vi "SaveLEDSettingsToFile.vi"(5 "Prefix":string="LEDSetting", 9 "Save?":bool, 10 "LED Color Ref":refnum<vi>, 11 "name or relative path":string) -> (3 "Saved Settings Path":path)   [LabVIEW 2015]
uses:
  <vilib>/Utility/sysdir.llb/System Directory Type.ctl
  <vilib>/Utility/file.llb/Write Delimited Spreadsheet (string).vi
panel:
  in  "LED Color":T1={"Hue"={110.52399131877658, 148.6727294921875}, "Sat"={34.78571428571429, 255.0}, "Val"={91.07142857142858, 255.0}} {"Hue" scale=0.0..255.0 scale format="%#_3g"}
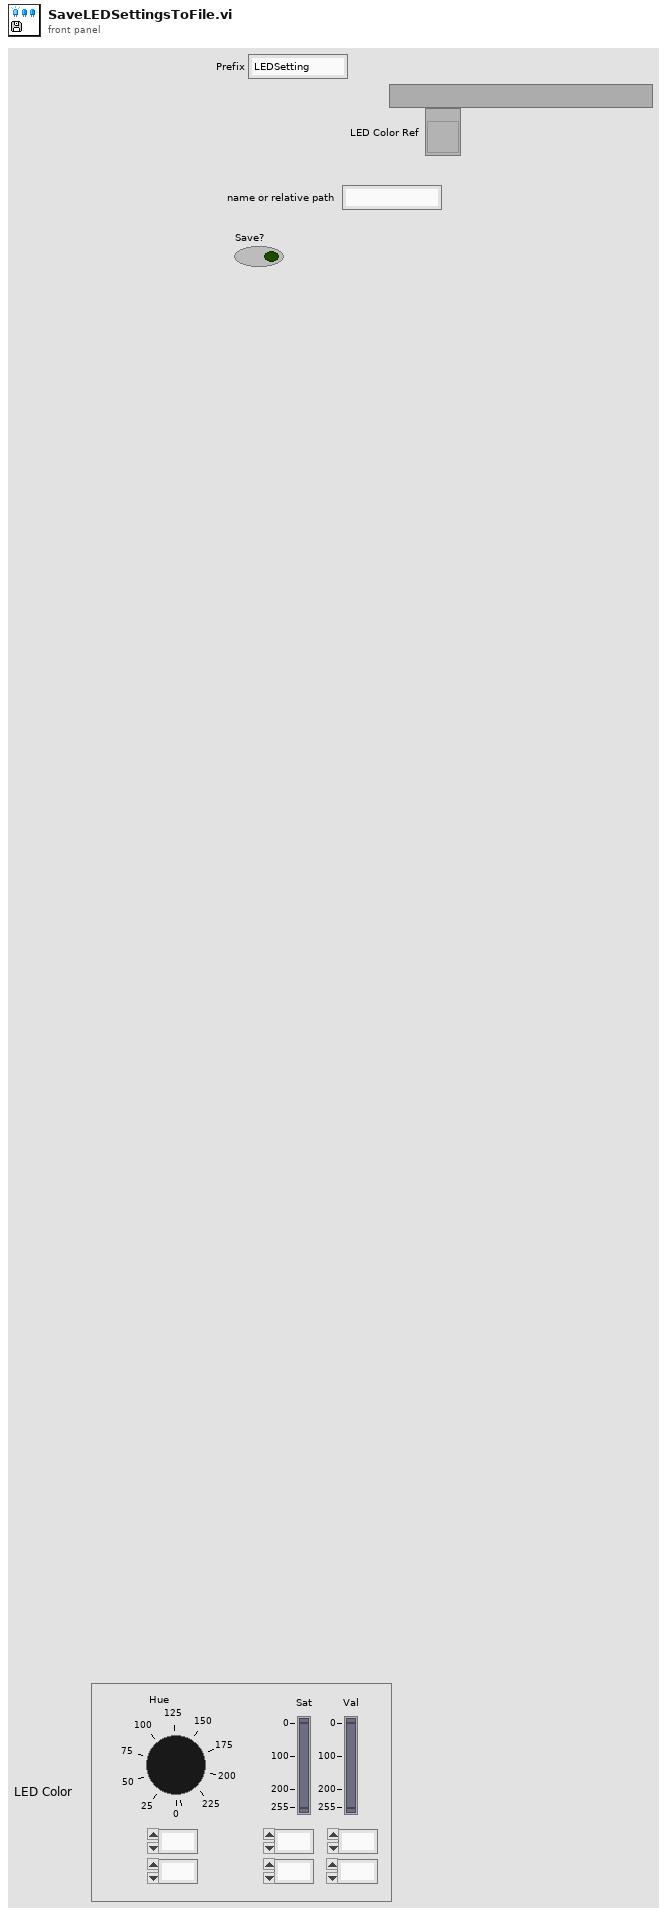
[diagram p1: front panel]
types:
  T1 = cluster{"Hue":cluster{dbl, dbl}, "Sat":cluster{dbl, dbl}, "Val":cluster{dbl, dbl}}
  T2 = typedef "System Directory Type.ctl" = i32
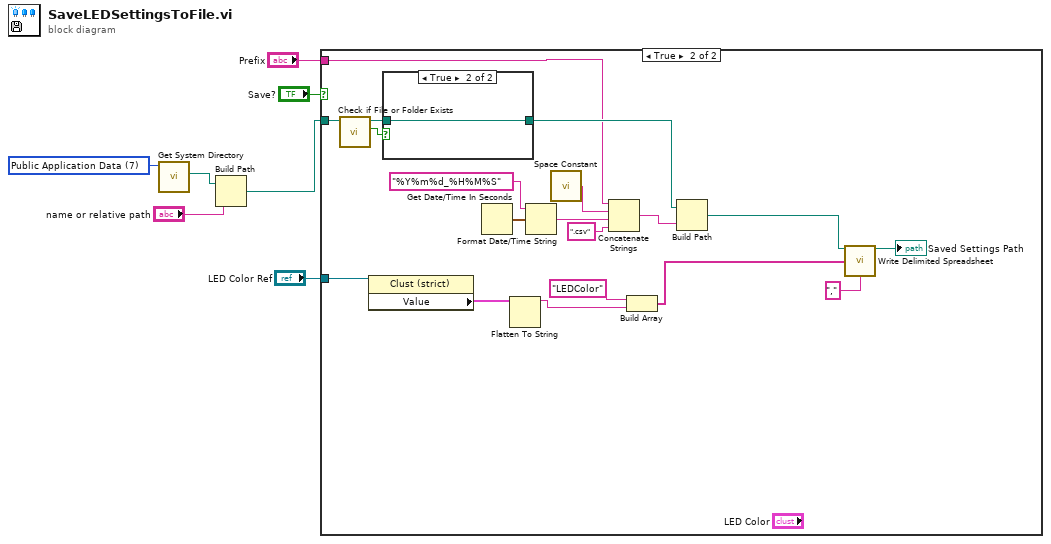
[diagram p0: block diagram]
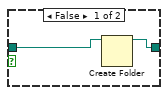
[diagram p3: hidden frame]
diagram:
  w4 = T2 7 items=["User Home"=0, "User Desktop"=1, "User Documents"=2, "User Application Data"=3, "User Preferences"=4, "User Temporary"=5, "Public Documents"=6, "Public Application Data"=7, "Public Preferences"=8, "Public Cache"=13, "System Core Libraries"=9, "System Installed Libraries"=10, "Application Files"=11, "Boot Volume Root"=12] ("system directory type")
  n1 = call <vilib>:"Get System Directory.vi"("system directory type"=w4) -> ("system directory"=w3:path)  [unwired: 10 in]
  n2 = Build Path(base path=w3, name or relative path="name or relative path") -> (appended path=w1:path)
  n3 = case shown="True" "Save?" {
    tunnel: w1 -> [_ w18]
    tunnel: "Prefix" -> [_ w14]
    tunnel: "LED Color Ref" -> [_ w12]
    frame False {
    }
    frame True {
      n4 = call <vilib>:"Check if File or Folder Exists.vi"("path"=w18) -> ("file or folder exists?"=w26:bool, "dup path"=w25:path)  [unwired: 8 in, 1 out]
      n5 = property class="Clust (strict)"(reference=w12) -> ("Value"=w11:T1)  [unwired: 1 in, 2 out]
      n6 = case shown="True" w26 {
        tunnel: w25 -> [w28 w29]
        tunnel: [w27 w29] -> w22
        frame False {
          n7 = Create Folder(path (use dialog)=w28) -> (created path=w27:path)  [unwired: 2 in, 2 out]
        }
        frame True {
        }
      }
      n8 = Get Date/Time In Seconds() -> (seconds since 1Jan1904=w24:timestamp)
      n9 = Flatten To String(anything=w11) -> (data string=w10:string)  [unwired: 3 in, 2 out]
      n10 = Format Date/Time String(time format string (%c)="%Y%m%d_%H%M%S", seconds (now)=w24) -> (date/time string=w21:string)  [unwired: 1 in]
      n11 = call <vilib>:"Space Constant.vi"() -> ("String"=w13:string)
      n12 = Concatenate Strings(w14, w13, w21, ".csv" ("string")) -> (w19:string)
      n13 = Build Array("LEDColor" ("element"), w10) -> (w8:string[])
      n14 = Build Path(base path=w22, name or relative path=w19) -> (appended path=w17:path)
      n15 = call-poly <vilib>:"Write Delimited Spreadsheet.vi"("file path (dialog if empty)"=w17, "1D data"=w8, "delimiter (\\t)"="," ("delimiter (\\t)")) -> ("new file path (Not A Path if cancelled)"=→"Saved Settings Path":path)  [unwired: 11 in, 1 out]
    }
  }
